vi "IndexAndScaleGeneratedData.vi"(6 "Type":T1, 7 "Lookup":variant, 8 "error in":errorcluster, 10 "ID":u32, 11 "VS Data":dbl[](array[numeric])) -> (0 "error out":errorcluster, 2 "Data":u8[](array[numeric]), 3 "VS Data":dbl[](array[numeric]))   [LabVIEW 2015, in "Diagnostics Addon Engine.lvlib"]
uses:
  Diagnostics Addon Engine.lvlib
  Shared/Types/MessageType Selector.ctl
  Shared/Types/Datatable Lookup Positions.ctl
  <vilib>/xnet/xnet.llb/XNET Convert (Signal to Frame Raw).vi
  Shared/SubVIs/GUID Lookup.vi
  Shared/Diagnostics Addon Shared.lvlib
  <vilib>/NI Veristand/Custom Device Tools/Custom Device Utility Library/Custom Device Utility Library.lvlib
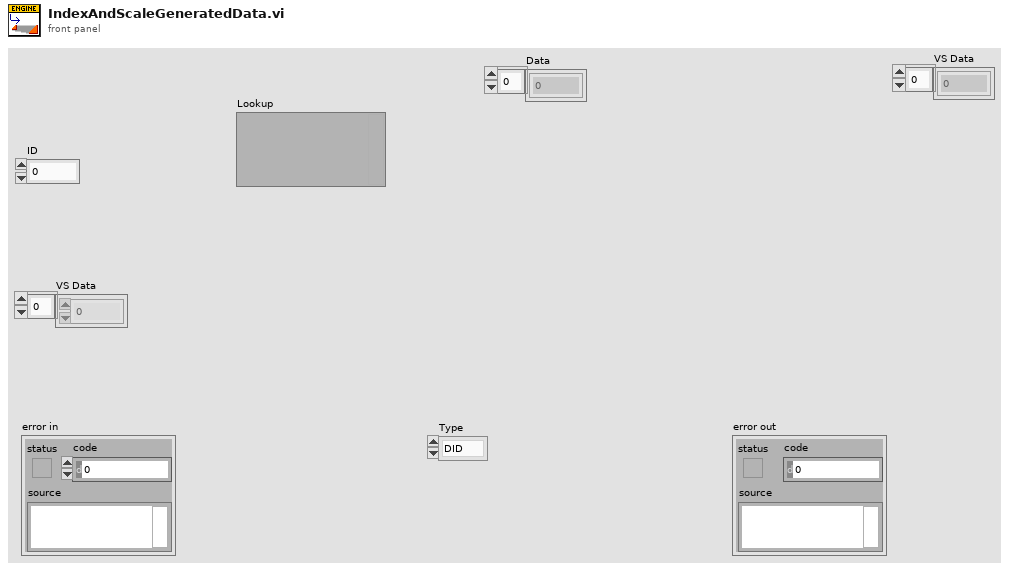
[diagram p1: front panel]
types:
  T1 = typedef "Diagnostics Addon Shared.lvlib/MessageType Selector.ctl" = enum16{"DID", "PID", "CPID", "Write Memory", "Read Memory", "DTC Control", "IO Cmd", "IO Resp", "Routine Start Cmd", "Routine Start Resp", "Routine Status Cmd", "Routine Status Resp", "Routine Stop Cmd", "Routine Stop Resp"}
  T2 = typedef "Diagnostics Addon Shared.lvlib/Datatable Lookup Positions.ctl" = cluster{"Offset":i32, "Length":i32, "ByteLength":u16}
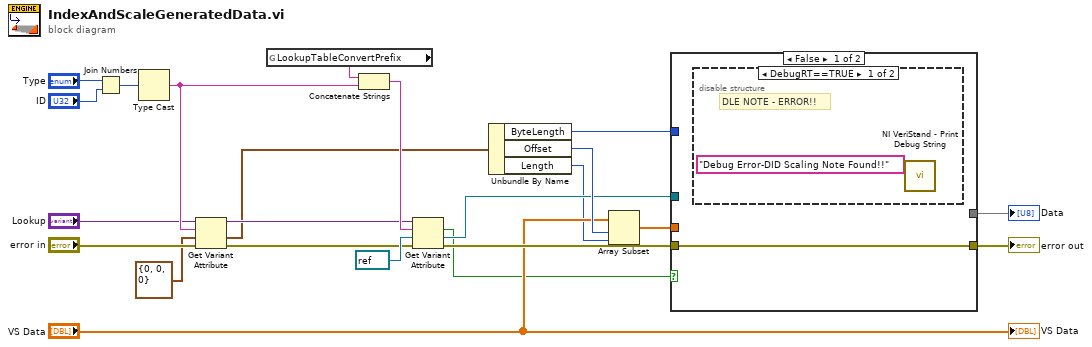
[diagram p0: block diagram]
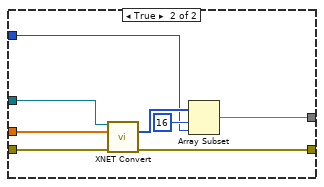
[diagram p3: hidden frame]
diagram:
  n1 = Join Numbers(hi="Type", lo="ID") -> ((hi.lo)=w2:u64)
  n2 = Type Cast(x=w2) -> (*(type *) &x=w17:string)  [unwired: 1 in]
  n3 = Get Variant Attribute(Variant="Lookup", name=w17, default value (empty Variant)=T2 {"Offset"=0, "Length"=0, "ByteLength"=0} ("cluster"), error in="error in") -> (duplicate Variant=w16:variant, value=w9:T2, error out=w18:errorcluster)  [unwired: 1 out]
  n4 = global read "GUID Lookup.vi" "LookupTableConvertPrefix"() -> (w19:string)
  n5 = Concatenate Strings(w19, w17) -> (w20:string)
  n6 = Get Variant Attribute(Variant=w16, name=w20, default value (empty Variant)=refnum<k21> refnum ("DID Conversion"), error in=w18) -> (found=w1:bool, value=w10:refnum<k21>, error out=w8:errorcluster)  [unwired: 1 out]
  n7 = Unbundle By Name(w9) -> ("ByteLength"=w13:u16, "Offset"=w12:i32, "Length"=w6:i32)
  n8 = Array Subset(array="VS Data", index=w12, length=w6) -> (w14:dbl[])
  n9 = case shown="False" w1 {
    tunnel: w8 -> [w24 w33]
    tunnel: [w24 w26] -> w5
    tunnel: w14 -> [_ w28]
    tunnel: w10 -> [_ w32]
    tunnel: w13 -> [_ w29]
    tunnel: [_ w27] -> w11
    frame False {
      n10 = disable-structure shown="DebugRT==TRUE" {
        frame condition #0 (active) {
          # "DLE NOTE - ERROR!!"
          n11 = call <vilib>:"NI VeriStand - Print Debug String.vi"("Message"="Debug Error-DID Scaling Note Found!!" ("Debug String")) -> ()  [unwired: 10 in, 1 out]
        }
        frame condition #1 {
        }
      }
    }
    frame True {
      n12 = call-poly <vilib>:"XNET Convert.vi"("session in"=w32, "signal data"=w28, "error in (no error)"=w33) -> ("frame data"=w31:u8[], "error out"=w26:errorcluster)  [unwired: 10 in, 1 out]
      n13 = Array Subset(array=w31, index=16, length=w29) -> (w27:u8[])
    }
  }
  "error out" <- w5
  "Data" <- w11
  "VS Data" <- "VS Data"
